vi "Read ID.vi"(8 "error in (no error)":errorcluster, 11 "Vaisala Probe in":refnum<class "Vaisala.lvclass">) -> (0 "error out":errorcluster, 2 "ID":string, 3 "Vaisala Probe out":refnum<class "Vaisala.lvclass">)   [LabVIEW 2014, in "Vaisala.lvclass"]
uses:
  Vaisala.lvclass
  Vaisala.lvclass/Vaisala.ctl
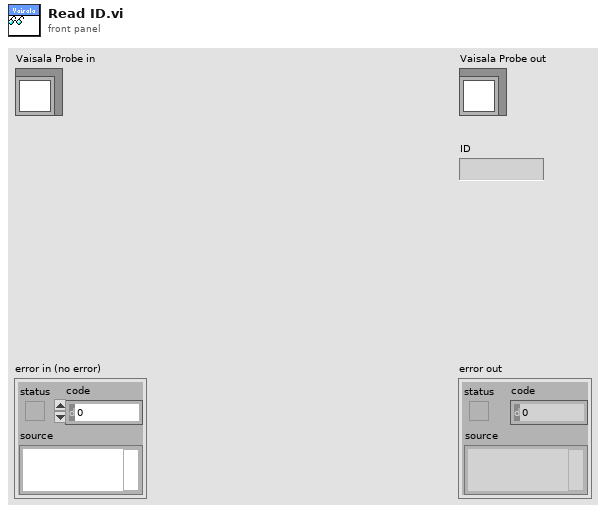
[diagram p1: front panel]
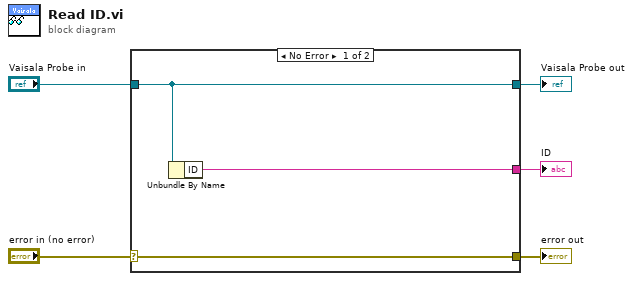
[diagram p0: block diagram]
diagram:
  n1 = case shown="No Error" "error in (no error)" {
    selector: "error in (no error)" -> [w8 w9]
    tunnel: [w8 w9] -> w4
    tunnel: [w7 w10] -> w2
    tunnel: "Vaisala Probe in" -> [w7 w10]
    tunnel: [w6 _] -> w1
    frame No Error {
      n2 = Unbundle By Name(w7) -> ("ID"=w6:string)
    }
    frame Error {
    }
  }
  "error out" <- w4
  "Vaisala Probe out" <- w2
  "ID" <- w1
